vi "Write BML OM.vi"(8 "error in (no error)":errorcluster, 10 "BML OM":T1, 11 "BML Pattern Creater in":refnum<class "BML Pattern Creater.lvclass">) -> (0 "error out":errorcluster, 3 "BML Pattern Creater out":refnum<class "BML Pattern Creater.lvclass">)   [LabVIEW 2018, in "BML Pattern Creater.lvlib" / "BML Pattern Creater.lvclass"]
uses:
  BML Pattern Creater.lvclass
  Ctls/OM - BML.ctl
  BML Pattern Creater.lvclass/BML Pattern Creater.ctl
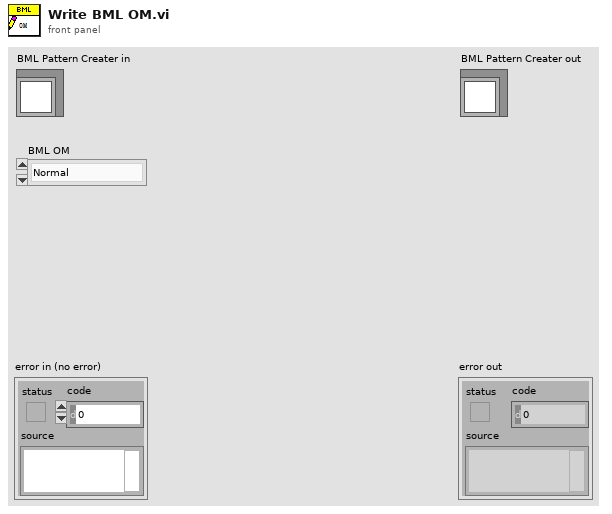
[diagram p1: front panel]
types:
  T1 = typedef "OM - BML.ctl" = enum16{"Normal", "ImmeEffect", "InitSlaveID", "LoadData"}
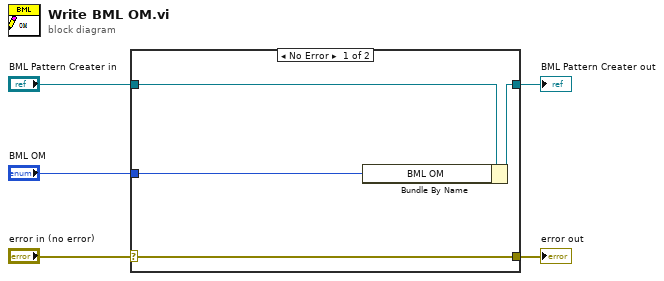
[diagram p0: block diagram]
diagram:
  n1 = case shown="No Error" "error in (no error)" {
    selector: "error in (no error)" -> [w9 w10]
    tunnel: [w9 w10] -> w4
    tunnel: [w7 w11] -> w2
    tunnel: "BML Pattern Creater in" -> [w8 w11]
    tunnel: "BML OM" -> [w6 _]
    frame No Error {
      n2 = Bundle By Name(cluster=w8, "BML OM"=w6) -> (w7:refnum<class "BML Pattern Creater.lvclass">)
    }
    frame Error {
    }
  }
  "error out" <- w4
  "BML Pattern Creater out" <- w2
